vi "Attempt camera connection.vi"(8 "error in (no error)":errorcluster, 11 "Camera session":T1) -> (0 "error out":errorcluster, 3 "Cam session Out":T1)   [LabVIEW 2020]
uses:
  <vilib>/userDefined/High Color/IMAQdx.ctl
  <vilib>/vision/driver/NI_Vision_Acquisition_Software.lvlib
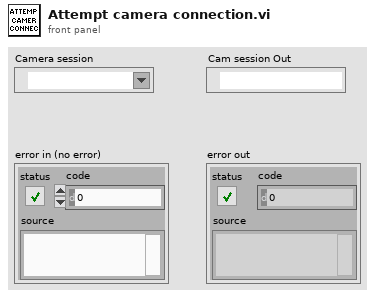
[diagram p1: front panel]
types:
  T1 = typedef "IMAQdx.ctl" = refnum<k21>
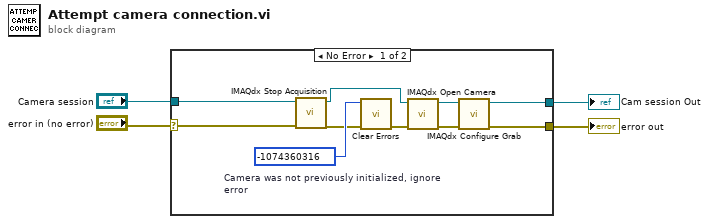
[diagram p0: block diagram]
diagram:
  n1 = case shown="No Error" "error in (no error)" {
    selector: "error in (no error)" -> [w13 w16]
    tunnel: "Camera session" -> [w14 w15]
    tunnel: [w12 w16] -> w2
    tunnel: [w5 w15] -> w1
    frame No Error {
      w9 = -1074360316  # Camera was not previously initialized, ignore error
      n2 = call <vilib>:"IMAQdx Stop Acquisition.vi"("error in"=w13, "Session In"=w14) -> ("error out"=w6:errorcluster, "Session Out"=w8:T1)  [unwired: 8 in]
      n3 = call <vilib>:"Clear Errors.vi"("error in (no error)"=w6, "specific error code to clear (0: all)"=w9) -> ("error out"=w7:errorcluster)  [unwired: 4 in, 1 out]
      n4 = call <vilib>:"IMAQdx Open Camera.vi"("error in"=w7, "Session In"=w8) -> ("error out"=w10:errorcluster, "Session Out"=w11:T1)  [unwired: 8 in]
      n5 = call <vilib>:"IMAQdx Configure Grab.vi"("error in"=w10, "Session In"=w11) -> ("error out"=w12:errorcluster, "Session Out"=w5:T1)  [unwired: 8 in]
    }
    frame Error {
    }
  }
  "error out" <- w2
  "Cam session Out" <- w1
